vi "SeperateArray.vi"(10 "mu08OutIndexCount":u8, 11 "mbfArrayIn":bool[](array[boolean])) -> (1 "mu08ArrayIndexFinalOut":u8[](array[numeric]), 3 "mu08ArrayIndexOutBuf":u8[](array[numeric]))   [LabVIEW 2011]
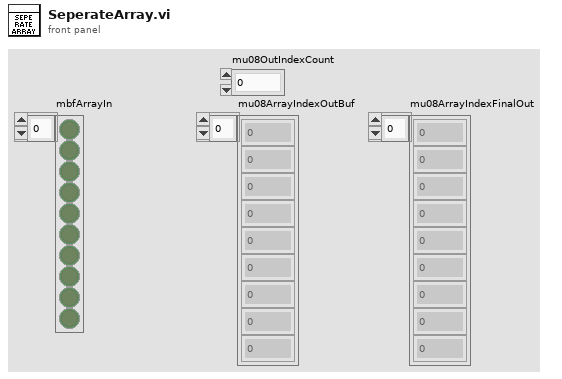
[diagram p1: front panel]
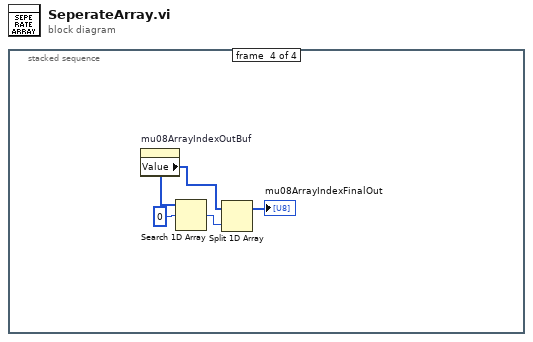
[diagram p0: block diagram]
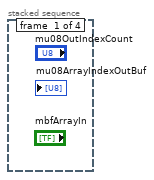
[diagram p2: hidden frame]
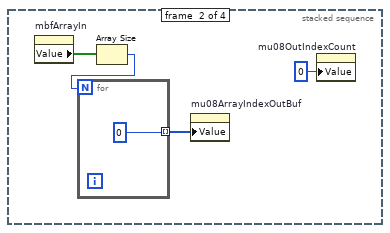
[diagram p3: hidden frame]
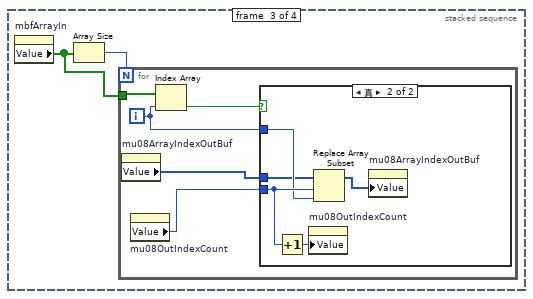
[diagram p4: hidden frame]
diagram:
  n1 = stacked-sequence {
    frame #0 {
    }
    frame #1 {
      n2 = property on="mbfArrayIn" class="Arr (严格)"() -> ("Value"=w4:bool[])  [unwired: 2 in, 2 out]
      n3 = Array Size(array=w4) -> (size(s)=w3:i32)
      n4 = for {
        N: w3 -> [_]
        tunnel: [0] -> w2 mode=indexing
      }
      n5 = property on="mu08ArrayIndexOutBuf" class="Arr (严格)"("Value"=w2) -> ()  [unwired: 2 in, 2 out]
      n6 = property on="mu08OutIndexCount" class="DigNum (严格)"("Value"=u8 0 ("mu08OutIndexCount")) -> ()  [unwired: 2 in, 2 out]
    }
    frame #2 {
      n7 = property on="mbfArrayIn" class="Arr (严格)"() -> ("Value"=w7:bool[])  [unwired: 2 in, 2 out]
      n8 = Array Size(array=w7) -> (size(s)=w6:i32)
      n9 = for {
        N: w6 -> [_]
        tunnel: w7 -> [w12]
        i -> [w10]
        n10 = property on="mu08ArrayIndexOutBuf" class="Arr (严格)"() -> ("Value"=w9:u8[])  [unwired: 2 in, 2 out]
        n11 = property on="mu08OutIndexCount" class="DigNum (严格)"() -> ("Value"=w8:u8)  [unwired: 2 in, 2 out]
        n12 = Index Array(array=w12, index=w10) -> (element=w11:bool)
        n13 = case shown="真" w11 {
          tunnel: w8 -> [_ w16]
          tunnel: w10 -> [_ w15]
          tunnel: w9 -> [_ w14]
          frame False {
          }
          frame True {
            n14 = Increment(x=w16) -> (x+1=w17:u8)
            n15 = property on="mu08OutIndexCount" class="DigNum (严格)"("Value"=w17) -> ()  [unwired: 2 in, 2 out]
            n16 = Replace Array Subset(array=w14, new element=w15, index=w16) -> (w13:u8[])
            n17 = property on="mu08ArrayIndexOutBuf" class="Arr (严格)"("Value"=w13) -> ()  [unwired: 2 in, 2 out]
          }
        }
      }
    }
    frame #3 {
      n18 = property on="mu08ArrayIndexOutBuf" class="Arr (严格)"() -> ("Value"=w20:u8[])  [unwired: 2 in, 2 out]
      n19 = Search 1D Array(1D array=w20, element=u8 0 ("元素")) -> (index of element=w19:i32)  [unwired: 1 in]
      n20 = Split 1D Array(array=w20, index=w19) -> (first subarray=→"mu08ArrayIndexFinalOut":u8[])  [unwired: 1 out]
    }
  }
